vi "Your_VI_Here.vi"(7 "Reset":bool, 10 "Hit?":bool) -> (2 "Shot\nCoordinates":T1)   [LabVIEW 2015]
doc: "Battleships algorithm VI. Replace the code on the block diagram with your algorithm for beating the game. Do not change the controls and indicators of this VI and do not modify the connector pane."
uses:
  TypDefs/Coordinates.ctl
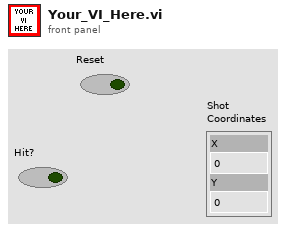
[diagram p1: front panel]
types:
  T1 = typedef "Coordinates.ctl" = cluster{"X":i32, "Y":i32}
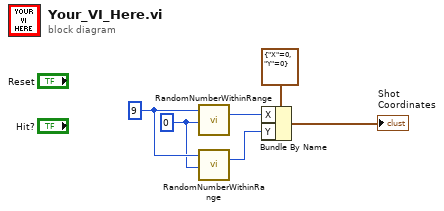
[diagram p0: block diagram]
diagram:
  w4 = 0 ("Low")
  w5 = 9 ("High")
  n1 = call "RandomNumberWithinRange.vi"("High"=w5, "Low"=w4) -> ("Random Number"=w3:i32)  [unwired: 25 in]
  n2 = call "RandomNumberWithinRange.vi"("High"=w5, "Low"=w4) -> ("Random Number"=w1:i32)  [unwired: 25 in]
  n3 = Bundle By Name(cluster=T1 {"X"=0, "Y"=0} ("Shot\nCoordinates"), "X"=w3, "Y"=w1) -> (→"Shot\nCoordinates":T1)
